vi "IC_GetVCDRange.vi"(0 "ICImagingControl3.IICImagingControl":refnum<k7>, 1 "Property":u16(ring) items=["Brightness", "Contrast", "Hue", "Saturation", "Sharpness", "Gamma", "Color Enable", "White Balance", "Backlight Compensation", "Gain", "Pan", "Tilt", "Roll", "Zoom", "Exposure", "Iris", "Focus", "Trigger Mode", "VCR Compatibility", "Signal Detected", "Testpattern", "GP IO", "Strobe"], 2 "Element ID":u16(ring) items=["Value", "Auto", "One Push", "Whitebalance Bue", "Whitebalance Red", "Auto Reference", "Trigger Polarity", "Trigger Mode", "Reset Value", "GP IO Input", "GP IO Output", "GP IO Write", "GP IO Read", "Strope Polarity", "Strobe Duration", "Strobe Delay"]) -> (4 "RangeMax":i32, 5 "ICImagingControl3.IICImagingControl 2":refnum<k7>, 6 "Available":bool, 7 "RangeMin":i32, 8 "Value":i32)   [LabVIEW 2015]
doc: "This VI sets a Switch for the passed VD Property"
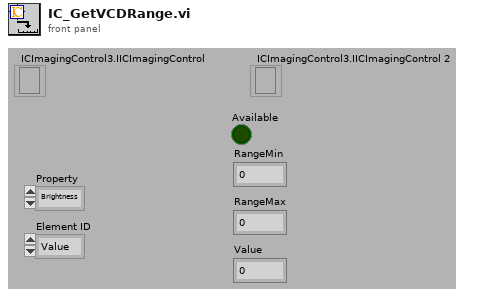
[diagram p1: front panel]
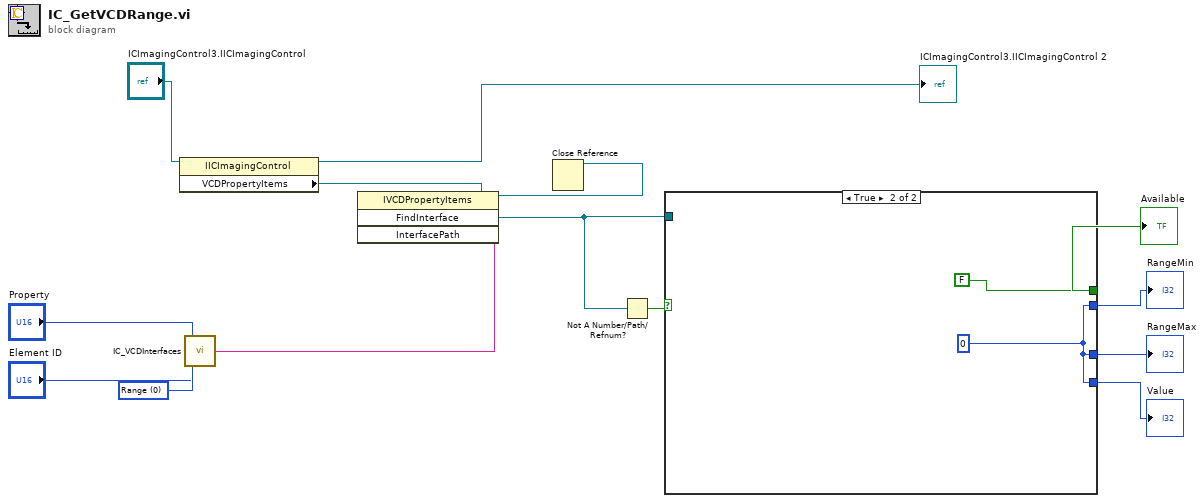
[diagram p0: block diagram]
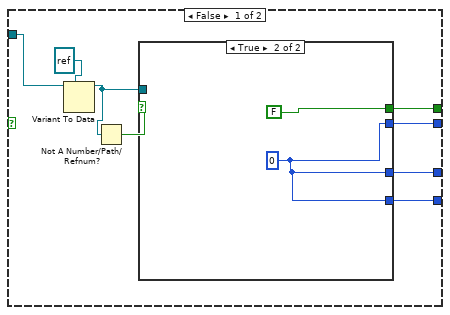
[diagram p2: hidden frame]
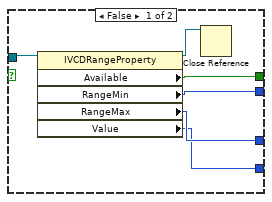
[diagram p3: hidden frame]
diagram:
  w9 = u16 0 items=["Range", "Switch", "Button", "Mapstrings", "Absolute Values"] ("Interface")
  n1 = property class="IICImagingControl"(reference="ICImagingControl3.IICImagingControl") -> (reference out=→"ICImagingControl3.IICImagingControl 2":refnum<k7>, "VCDPropertyItems"=w11:refnum<k7>)  [unwired: 1 in, 1 out]
  n2 = call "IC_VCDInterfaces.vi"("Interface"=w9, "Element ID"="Element ID", "Property"="Property") -> ("Interface Path"=w10:string)
  n3 = invoke class="IVCDPropertyItems" method="FindInterface"(reference=w11, "InterfacePath"=w10) -> (reference out=w12:refnum<k7>, "FindInterface"=w6:refnum<k7>)  [unwired: 2 in, 2 out]
  n4 = Close Reference(reference=w12) -> ()  [unwired: 1 in, 1 out]
  n5 = Not A Number/Path/Refnum?(number/path/refnum=w6) -> (NaN/Path/Refnum?=w5:bool)
  n6 = case shown="True" w5 {
    tunnel: w6 -> [w19 _]
    tunnel: [w18 FALSE] -> w4
    tunnel: [w17 w31] -> w3
    tunnel: [w15 w31] -> w2
    tunnel: [w16 w31] -> w1
    frame False {
      n7 = Variant To Data(type=refnum<k7> refnum ("ICImagingControl3.IVCDRangeProperty"), Variant=w19) -> (data=w21:refnum<k7>)  [unwired: 1 in, 1 out]
      n8 = Not A Number/Path/Refnum?(number/path/refnum=w21) -> (NaN/Path/Refnum?=w22:bool)
      n9 = case shown="True" w22 {
        tunnel: w21 -> [w27 _]
        tunnel: [w26 FALSE] -> w18
        tunnel: [w25 w30] -> w17
        tunnel: [w23 w30] -> w16
        tunnel: [w24 w30] -> w15
        frame False {
          n10 = property class="IVCDRangeProperty"(reference=w27) -> (reference out=w28:refnum<k7>, "Available"=w26:bool, "RangeMin"=w25:i32, "RangeMax"=w24:i32, "Value"=w23:i32)  [unwired: 1 in, 1 out]
          n11 = Close Reference(reference=w28) -> ()  [unwired: 1 in, 1 out]
        }
        frame True {
          w30 = 0
        }
      }
    }
    frame True {
      w31 = 0
    }
  }
  "Available" <- w4
  "RangeMin" <- w3
  "RangeMax" <- w2
  "Value" <- w1
